vi "StringThing.vi"(7 "Signal Name":string, 8 "Input":dbl, 11 "Carry":string) -> (3 "Output":string)   [LabVIEW 2016]
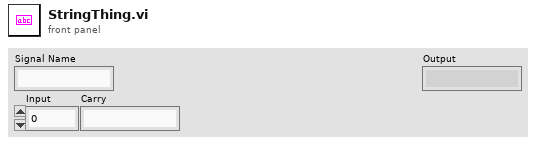
[diagram p1: front panel]
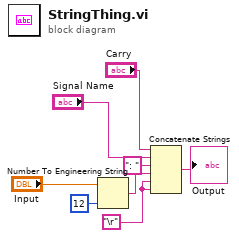
[diagram p0: block diagram]
diagram:
  w1 = "\r"
  n1 = Number To Engineering String(2:i16 12 ("precision (6)"), 4:"Input") -> (0:w8:string)  [unwired: 2 in]
  n2 = Concatenate Strings("Carry", "Signal Name", ": " ("string"), w8, w1, w1) -> (→"Output":string)
